vi "Mouse Coords to Chess Position.vi"(10 "coords":T1) -> (1 "column":i32, 2 "row":i32)   [LabVIEW 2018, in "Othello.xctl"]
doc: "本VI是为《我和LabVIEW》一书编写的示例。\n关于本书的介绍请参考网页：\nhttp://ruanqizhen.spaces.live.com/blog/cns!5852D4F797C53FB6!4310.entry"
uses:
  Othello.xctl
  <vilib>/Utility/miscctls.llb/LVPoint32TypeDef.ctl
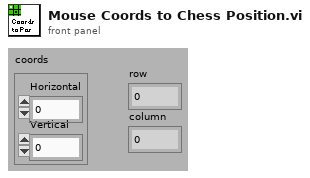
[diagram p1: front panel]
types:
  T1 = typedef "LVPoint32TypeDef.ctl" = cluster{"Horizontal":i32, "Vertical":i32}
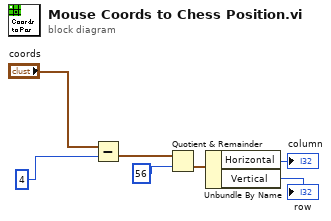
[diagram p0: block diagram]
diagram:
  n1 = Subtract(x="coords", y=4 ("Horizontal")) -> (x-y=w5:T1)
  n2 = Quotient & Remainder(x=w5, y=56 ("Horizontal")) -> (floor(x/y)=w1:T1)  [unwired: 1 out]
  n3 = Unbundle By Name(w1) -> ("Horizontal"=→"column":i32, "Vertical"=→"row":i32)
